vi "MdsDescrSingle2D.vi"(0 "Value In":sgl[][](array[numeric])) -> (1 "DescrId":i32, 2 "ValueOut":sgl[][](array[numeric]))   [LabVIEW 2011]
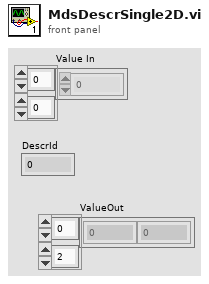
[diagram p1: front panel]
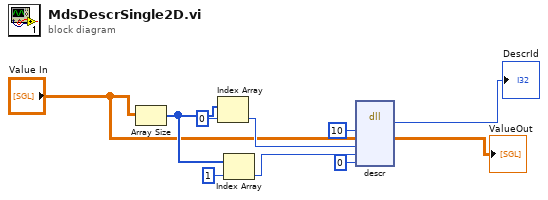
[diagram p0: block diagram]
diagram:
  n1 = Array Size(array="Value In") -> (size(s)=w9:i32[])
  n2 = Index Array(array=w9, index=0) -> (element=w7:i32)
  n3 = Index Array(array=w9, index=1) -> (element=w6:i32)
  n4 = dll-call lib="MdsLib" fn="descr"("dtype"=10, "value"="Value In", "dim0"=w7, "dim1"=w6, "endarg"=0) -> ("return type"=→"DescrId":i32, "value"=→"ValueOut":sgl[][])  [unwired: 7 in, 2 out]
